vi "Gradient_Search_v12 (SubVI).vi"(0 "Speed factor":dbl=5.0, 1 "Max velocity":dbl=5.0, 2 "ML":dbl=0.1, 3 "Min Radius":dbl=0.5, 4 "Max Radius":dbl=2.0, 5 "GS Frequency":dbl=2.5, 6 "Max. dir. changes":i32=50, 7 "error in (no error)":errorcluster, 8 "Analog Input":i32, 9 "Run?":bool, 10 "System no.":i32, 11 "Tracking":bool) -> (19 "error out":errorcluster)   [LabVIEW 2023]
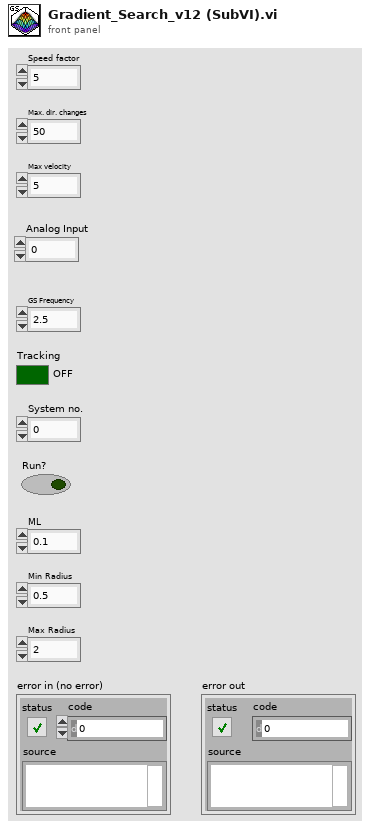
[diagram p1: front panel]
types:
  T1 = cluster{"Min amplitude":dbl, "Set min. amplitude?":bool, "Max amplitude":dbl, "Set max. amplitude?":bool}
  T2 = cluster{"Set max. dir. changes?":bool, "Max. dir. changes":i32}
  T3 = cluster{"Set speed factor?":bool, "Speed factor":dbl}
  T4 = cluster{"Set max. velocity?":bool, "Max velocity":dbl}
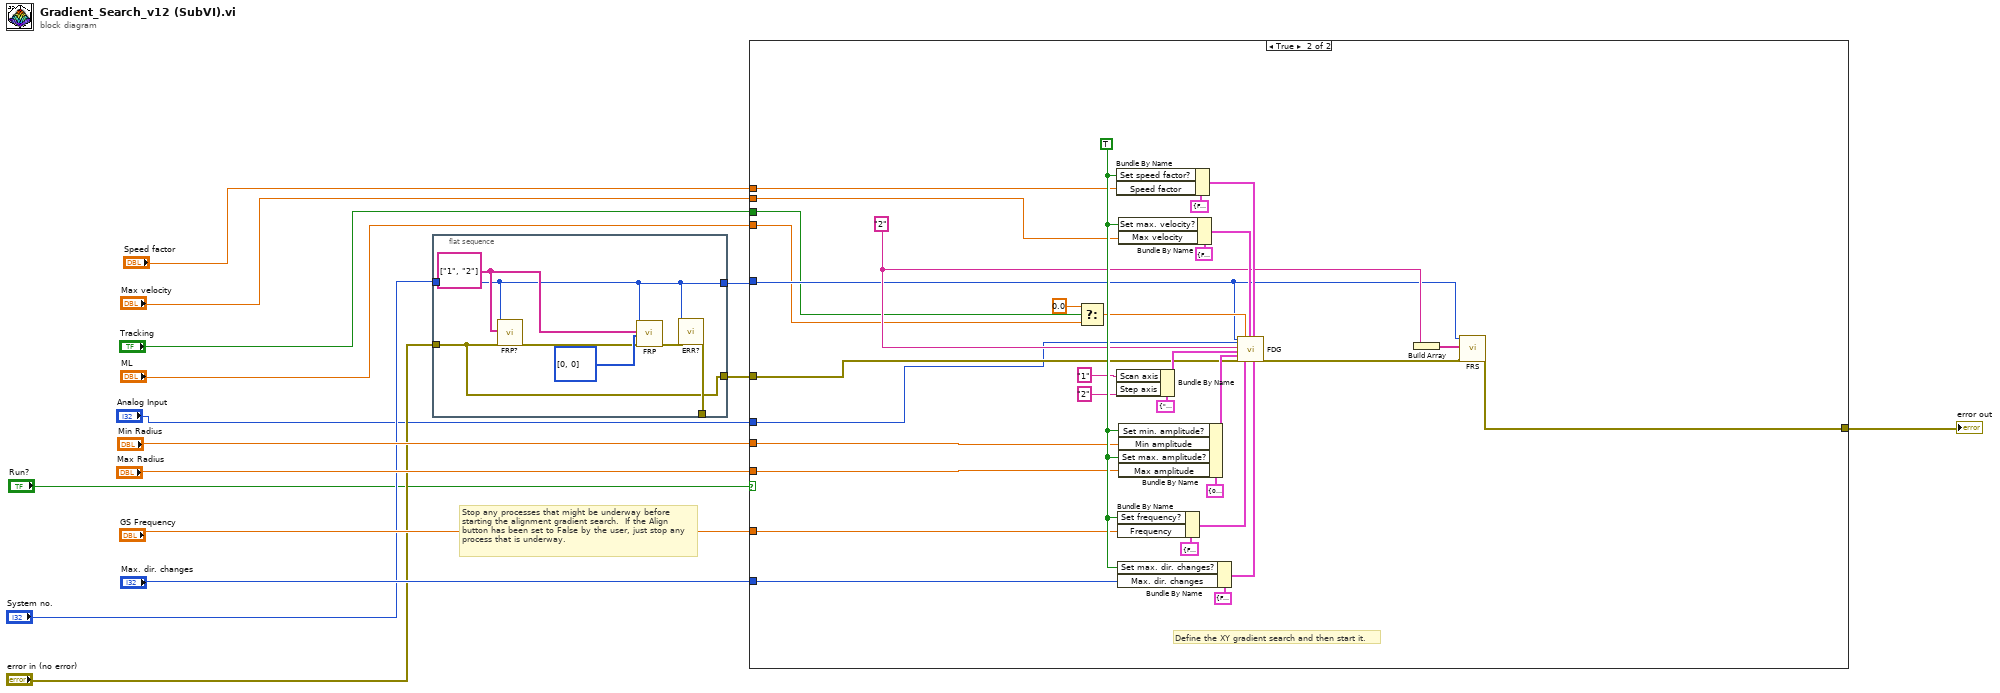
[diagram p0: block diagram]
diagram:
  # "Stop any processes that might be underway before\nstarting the alignment gradient search.  If the Align\nbutton has been set to False by the user, just stop any\nprocess that is underway."
  n1 = flat-sequence {
    tunnel: "error in (no error)" -> [w17]
    tunnel: "System no." -> [w16]
    tunnel: [w18] -> _
    tunnel: [w17] -> w7
    tunnel: [w16] -> w5
    frame #0 {
      w20 = string[] ["1", "2"] ("Routinename")
      n2 = call "FRP?.vi"("System no."=w16, "Routines to query"=w20, "error in"=w17) -> ("error out"=w19:errorcluster)  [unwired: 15 in, 1 out]
      n3 = call "FRP.vi"("System no."=w16, "Routinename"=w20, "Option"=i32[] [0, 0], "error in"=w19) -> ("error out"=w22:errorcluster)  [unwired: 15 in]
      n4 = call "ERR?.vi"("System no."=w16, "error in"=w22) -> ("error out"=w18:errorcluster)  [unwired: 16 in, 1 out]
    }
  }
  n5 = case shown="True" "Run?" {
    tunnel: w7 -> [w23 w33]
    tunnel: [w23 w37] -> w2
    tunnel: w5 -> [_ w34]
    tunnel: "GS Frequency" -> [_ w32]
    tunnel: "Max. dir. changes" -> [_ w31]
    tunnel: "Min Radius" -> [_ w30]
    tunnel: "Max Radius" -> [_ w29]
    tunnel: "Analog Input" -> [_ w28]
    tunnel: "ML" -> [_ w27]
    tunnel: "Tracking" -> [_ w26]
    tunnel: "Max velocity" -> [_ w25]
    tunnel: "Speed factor" -> [_ w24]
    frame False {
    }
    frame True {
      w40 = "2" ("String")
      w43 = TRUE ("Set speed factor?")
      # "Define the XY gradient search and then start it."
      n6 = Select(t=0.0, s=w26, f=w27) -> (s? t:f=w42:dbl)
      n7 = Bundle By Name(cluster=T3 {"Set speed factor?"=FALSE, "Speed factor"=0.25} ("Speed factor settings"), "Set speed factor?"=w43, "Speed factor"=w24) -> (w52:T3)
      n8 = Bundle By Name(cluster=cluster{"Scan axis":string, "Step axis":string} {"Scan axis"="", "Step axis"=""} ("Axis settings"), "Scan axis"="1" ("String"), "Step axis"="2" ("String")) -> (w46:cluster{"Scan axis":string, "Step axis":string})
      n9 = Bundle By Name(cluster=cluster{"Set frequency?":bool, "Frequency":dbl} {"Set frequency?"=FALSE, "Frequency"=10.0} ("Frequency settings"), "Set frequency?"=w43, "Frequency"=w32) -> (w50:cluster{"Set frequency?":bool, "Frequency":dbl})
      n10 = Bundle By Name(cluster=T2 {"Set max. dir. changes?"=FALSE, "Max. dir. changes"=10} ("Max. direction changes settings"), "Set max. dir. changes?"=w43, "Max. dir. changes"=w31) -> (w48:T2)
      n11 = Bundle By Name(cluster=T4 {"Set max. velocity?"=FALSE, "Max velocity"=4.0} ("Velocity settings"), "Set max. velocity?"=w43, "Max velocity"=w25) -> (w54:T4)
      n12 = Bundle By Name(cluster=T1 {"Min amplitude"=0.4, "Set min. amplitude?"=FALSE, "Max amplitude"=0.8, "Set max. amplitude?"=FALSE} ("Amplitude settings"), "Set min. amplitude?"=w43, "Min amplitude"=w30, "Set max. amplitude?"=w43, "Max amplitude"=w29) -> (w44:T1)
      n13 = call "FDG.vi"("System no."=w34, "Board"=w28, "Routinename"=w40, "Axis settings"=w46, "Amplitude settings"=w44, "error in"=w33, "Minimum Level"=w42, "Frequency settings"=w50, "Velocity settings"=w54, "Speed factor settings"=w52, "Max. direction changes settings"=w48) -> ("error out"=w38:errorcluster)  [unwired: 1 in, 7 out]
      n14 = Build Array(w40) -> (w39:string[])
      n15 = call "FRS.vi"("System no."=w34, "Routines to start"=w39, "error in"=w38) -> ("error out"=w37:errorcluster)  [unwired: 16 in]
    }
  }
  "error out" <- w2
